vi "Unlock_File_manual.vi"() -> ()   [LabVIEW 2010]
panel:
  out "No of Files":i32
  out "Files Processed":i32
  out "Path":path
  in  "Mode":enum16{"Single File", "All Files inside Folder"}(ring)
  in  "Lock File":bool
  out "File Path":path
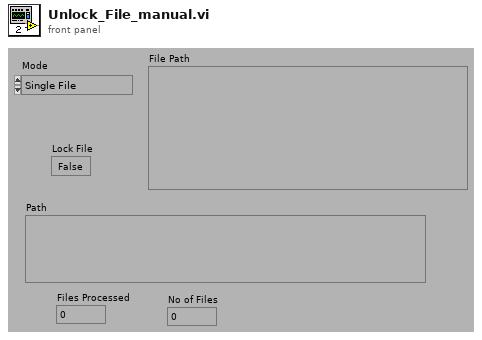
[diagram p1: front panel]
types:
  T1 = enum32{"existing file", "new file", "new or existing file", "existing dir", "new dir", "new or existing dir", "existing file (use LLBs)", "new file (use LLBs)", "new or existing file (use LLBs)", "new or existing file or directory (use LLBs)"}
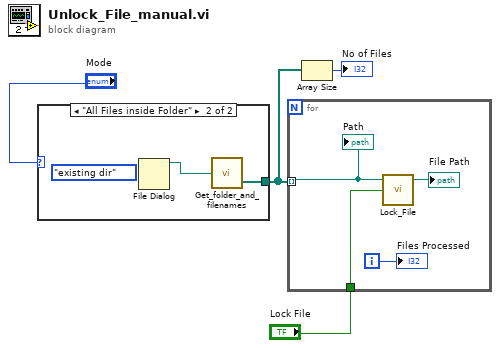
[diagram p0: block diagram]
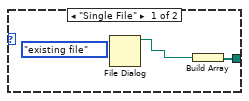
[diagram p2: hidden frame]
diagram:
  n1 = case shown="\"All Files inside Folder\"" "Mode" {
    tunnel: [w5 w8] -> w2
    frame "Single File" {
      (unwired) T1."existing file" ("select mode (2)")
      n2 = File Dialog() -> (3:w6:path)  [unwired: 7 in, 3 out]
      n3 = Build Array(w6) -> (w5:path[])
    }
    frame "All Files inside Folder" {
      (unwired) T1."existing dir" ("select mode (2)")
      n4 = File Dialog() -> (3:w7:path)  [unwired: 7 in, 3 out]
      n5 = call "Get_folder_and_filenames.vi"("file path (dialog if empty)"=w7) -> ("Files"=w8:path[])  [unwired: 1 out]
    }
  }
  n6 = for {
    tunnel: w2 -> [w12] mode=indexing
    tunnel: "Lock File" -> [w11]
    i -> [w9]
    n7 = call "Lock_File.vi"("Lock File"=w11, "path"=w12) -> ("dup path"=→"File Path":path)  [unwired: 2 in, 1 out]
    "Path" <- w12
    "Files Processed" <- w9
  }
  n8 = Array Size(array=w2) -> (size(s)=→"No of Files":i32)
